vi "Delete_Subscriber.vi"(8 "error in (no error)":errorcluster, 10 "N":i32=1 min=1 max=20, 11 "Delete_Subscriber":string="//Delete_subscriber") -> (0 "error out":errorcluster, 3 "Output String":string)   [LabVIEW 2021]
uses:
  Controls/TCP_FGV.ctl
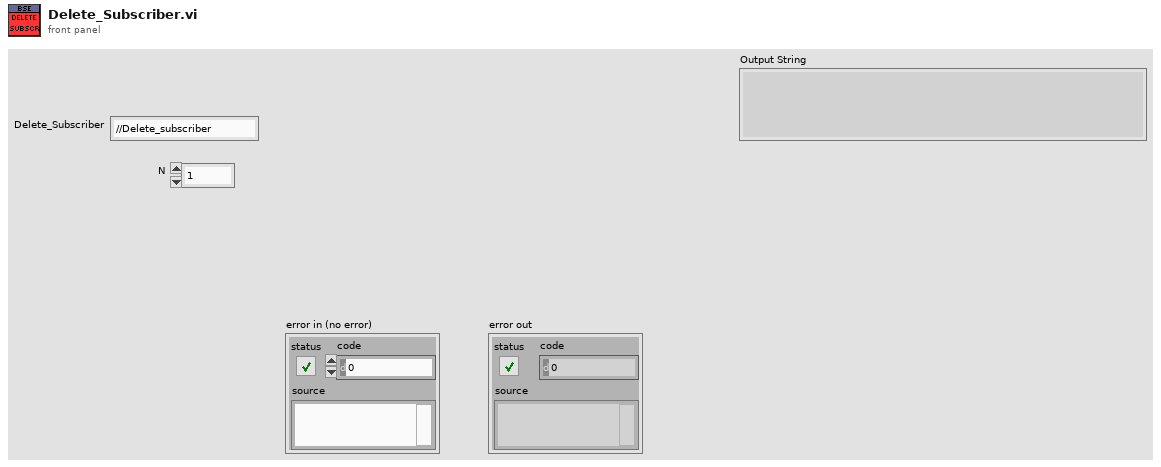
[diagram p1: front panel]
types:
  T1 = typedef "TCP_FGV.ctl" = enum16{"Open", "Read", "Write", "Close"}
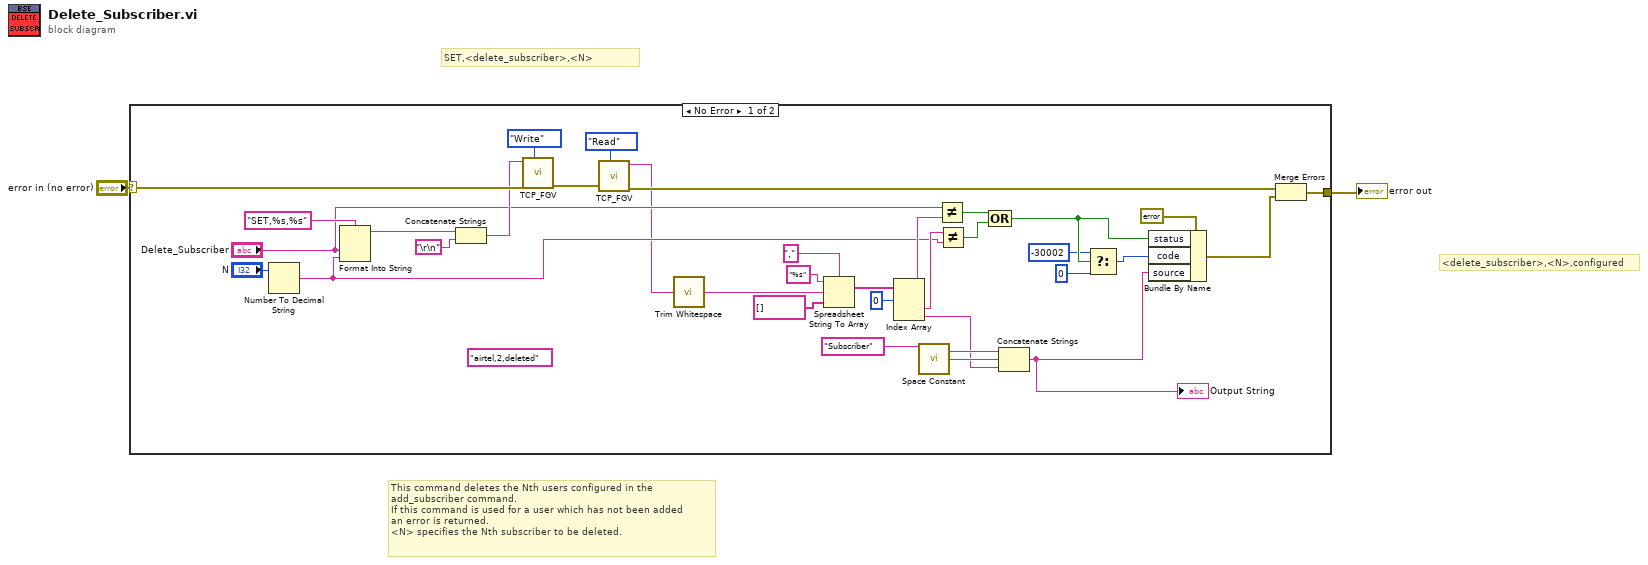
[diagram p0: block diagram]
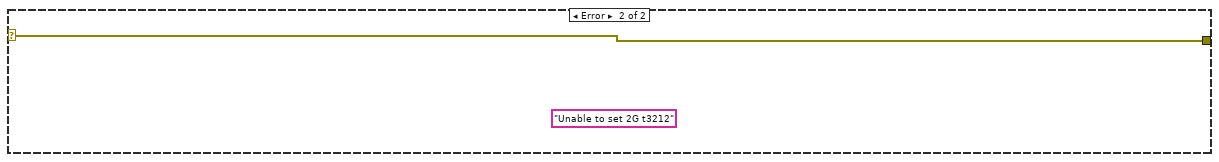
[diagram p2: hidden frame]
diagram:
  # "This command deletes the Nth users configured in the \nadd_subscriber command.   \nIf this command is used for a user which has not been added \nan error is returned.  \n<N> specifies the Nth subscriber to be deleted."
  # "SET,<delete_subscriber>,<N>"
  # "<delete_subscriber>,<N>,configured"
  n1 = case shown="No Error" "error in (no error)" {
    selector: "error in (no error)" -> [w35 w37]
    tunnel: [w19 w37] -> w1
    frame No Error {
      (unwired) "airtel,2,deleted" ("format string")
      n2 = Number To Decimal String(number="N") -> (decimal integer string=w9:string)  [unwired: 1 in]
      n3 = Format Into String(format string="SET,%s,%s", "Delete_Subscriber", w9) -> (resulting string=w15:string)  [unwired: 2 in, 1 out]
      n4 = Concatenate Strings(w15, "\r\n") -> (w14:string)
      n5 = call "TCP_FGV.vi"("Command"=w14, "error in (no error)"=w35, "Operation"=TCP_FGV."Write") -> ("error out"=w20:errorcluster)  [unwired: 6 in, 1 out]
      n6 = call "TCP_FGV.vi"("error in (no error)"=w20, "Operation"=TCP_FGV."Read") -> ("Data Out"=w3:string, "error out"=w22:errorcluster)  [unwired: 7 in]
      n7 = call <vilib>:"Trim Whitespace.vi"("string"=w3) -> ("trimmed string"=w32:string)  [unwired: 1 in]
      n8 = Spreadsheet String To Array(delimiter (Tab)=",", format string="%s", spreadsheet string=w32, array type (2D Dbl)=string[] []) -> (array=w29:string[])
      n9 = Index Array(array=w29, index #1=0 ("index")) -> (element #1=w11:string, element #2=w30:string, element #3=w6:string)  [unwired: 2 in]
      n10 = call <vilib>:"Space Constant.vi"() -> ("String"=w8:string)
      n11 = Not Equal?(x="Delete_Subscriber", y=w11) -> (x != y?=w12:bool)
      n12 = Not Equal?(x=w30, y=w9) -> (x != y?=w31:bool)
      n13 = Compound Arithmetic op=OR(w12, w31) -> (w33:bool)
      n14 = Concatenate Strings("Subscriber" ("format string"), w8, w6) -> (w18:string)
      "Output String" <- w18
      n15 = Select(t=-30002 ("code"), s=w33, f=0 ("code")) -> (s? t:f=w34:i32)
      n16 = Bundle By Name(cluster=errorcluster {"status"=FALSE, "code"=0, "source"=""} ("error constant"), "status"=w33, "code"=w34, "source"=w18) -> (w21:errorcluster)
      n17 = Merge Errors(w22, w21) -> (w19:errorcluster)
    }
    frame Error {
      (unwired) "Unable to set 2G t3212" ("source")
    }
  }
  "error out" <- w1
